vi "DEMO.vi"   [LabVIEW 2018, in "VXMx2.lvclass"]
uses:
  VXMx2.lvclass
  <instrlib>/Velmex VXM/Public/VXM Axis.ctl
  <instrlib>/Velmex VXM/Velmex VXM.lvlib
types:
  T1 = typedef "Velmex VXM.lvlib/VXM Axis.ctl" = u16
  T2 = cluster{"X mm/step":dbl, "Y mm/step":dbl, "Z mm/step":dbl, "T deg/step":dbl}
  T3 = cluster{"X step":dbl, "Y step":dbl, "Z step":dbl, "T step":dbl}
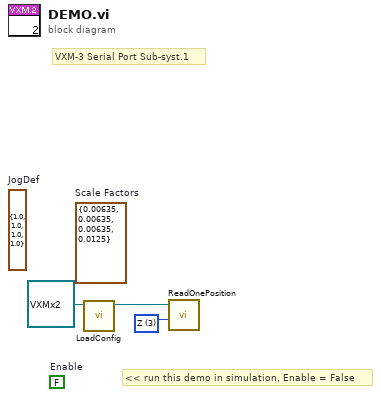
[diagram p0: block diagram]
diagram:
  w1 = T1 3 items=["X"=1, "Y"=2, "Z"=3, "T"=4] ("Axis (1..4)")
  (unwired) T2 {"X mm/step"=0.00635, "Y mm/step"=0.00635, "Z mm/step"=0.00635, "T deg/step"=0.0125}  # Scale Factors
  (unwired) T3 {"X step"=1.0, "Y step"=1.0, "Z step"=1.0, "T step"=1.0}  # JogDef
  (unwired) FALSE  # Enable
  # "VXM-3 Serial Port Sub-syst.1"
  # "<< run this demo in simulation, Enable = False"
  n1 = call "LoadConfig.vi"("VXMx2 in"=refnum<class "VXMx2.lvclass"> refnum) -> ("VXMx2 out"=w3:refnum<class "VXMx2.lvclass">)  [unwired: 9 in, 1 out]
  n2 = call "ReadOnePosition.vi"("Axis (1..4)"=w1, "VXMx2 in"=w3) -> ()  [unwired: 7 in, 3 out]
